vi "Block_string_to_array.vi"(0 "transmitted string":string, 1 "check size":i32=2) -> (2 "array of velocity data":u16[](array[numeric])=[2626, 2594, 18746, 18693, 2316, 18730, 2437, 2761, 2804, 2801, 19385, 19357, 19268, 2851, 2908, 2825, 2764, 2330, 2900, 2646, 2894, 2507, 2686, 2790, 2496, 1974, 2403, 2684, 2664, 2265, 2556, 2715, 2757, 2759, 2679, 2471, 2615, 2995, 2646, 2709, 2829, 2705, 2622, 2794, 2619, 2822, 2488, 19008, 2829, 2579, 18650, 2403, 2882, 2631, 2916, 2178, 18880, 2896, 19222, 18560, 17309, 17024, 18176, 17181, 18147, 3188, 2818, 2470, 2734, 2588, 2525, 2572, 19212, 2572, 2769, 2659, 2198, 2162, 2732, 19241, 3019, 3003, 2818, 2922, 2450, 2964, 2601, 18877, 18867, 2493, 2766, 2641, 2535, 2997, 2897, 2573, 2944, 17053, 17037, 17152, 19229, 19683, 2742, 2648, 2667, 2815, 3157, 19334, 2385, 2786, 19014, 2473, 3086, 3033, 18574, 18583, 18580, 19242, 2695, 2715, 3029, 18620, 2752, 2856, 2798, 2390, 2888, 3016, 2910, 2814, 18615, 2564, 18900, 2828, 3049, 18442, 2352, 2820, 2202, 2170, 2617, 19249, 2812, 2797, 2593, 2708, 19442, 3176, 3328, 3273, 2871, 2550, 2712, 19318, 2385, 19036, 2696, 2840, 2957, 2741, 2988, 2835, 18706, 2355, 19091, 2169, 2664, 2622, 2650, 18876, 2649, 2566, 18048, 2376, 2424, 3230, 2645, 2504, 2860, 2747, 2758, 2699, 2298, 2567, 2513, 2231, 2268, 2287, 2539, 2667, 2499, 2485, 2678, 2885, 2896, 2859, 3098, 2993, 3005, 19208] format="%.0x", 3 "transmission check":u16=400, 4 "transmission okay":bool=TRUE)   [LabVIEW 2010]
panel:
  out "trans check":string
  out "Block length":i32=200
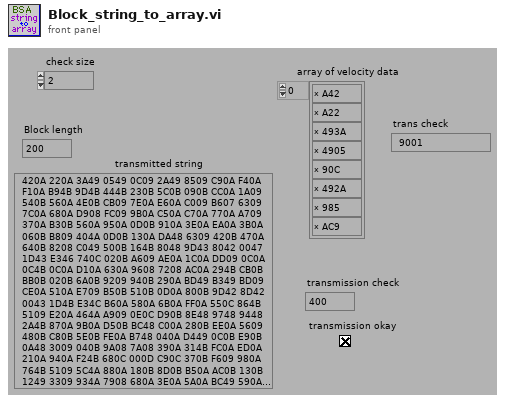
[diagram p1: front panel]
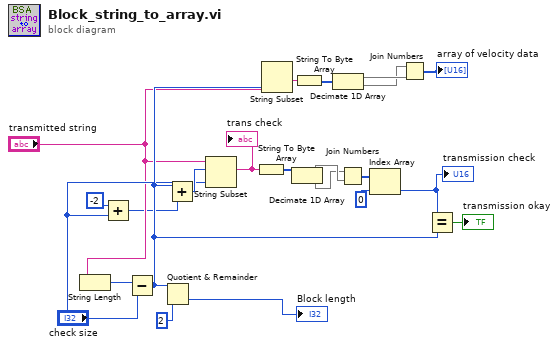
[diagram p0: block diagram]
diagram:
  n1 = String Length(string="transmitted string") -> (length=w19:i32)
  n2 = Add(x=-2, y="check size") -> (x+y=w2:i32)
  n3 = Subtract(x=w19, y="check size") -> (x-y=w8:i32)
  n4 = Quotient & Remainder(x=w8, y=2) -> (floor(x/y)=→"Block length":i32)  [unwired: 1 out]
  n5 = Add(x=w8, y=w2) -> (x+y=w7:i32)
  n6 = String Subset(string="transmitted string", offset (0)=w7, length (rest)="check size") -> (substring=w17:string)
  "trans check" <- w17
  n7 = String To Byte Array(string=w17) -> (unsigned byte array=w16:u8[])
  n8 = String Subset(string="transmitted string", length (rest)=w8) -> (substring=w18:string)  [unwired: 1 out]
  n9 = Decimate 1D Array(w16) -> (w6:u8[], w5:u8[])
  n10 = String To Byte Array(string=w18) -> (unsigned byte array=w21:u8[])
  n11 = Decimate 1D Array(w21) -> (w11:u8[], w10:u8[])
  n12 = Join Numbers(hi=w5, lo=w6) -> ((hi.lo)=w15:u16[])
  n13 = Index Array(array=w15, index=0) -> (element=w13:u16)
  "transmission check" <- w13
  n14 = Join Numbers(hi=w10, lo=w11) -> ((hi.lo)=→"array of velocity data":u16[])
  n15 = Equal?(x=w13, y=w8) -> (x = y?=→"transmission okay":bool)
